vi "Bead threshold manual adjust.vi"(8 "error in (no error)":errorcluster, 9 "Range":cluster{"Lower value":sgl, "Upper value":sgl}={"Lower value"=40.0, "Upper value"=255.0}, 10 "Particle Filter Image":T1, 11 "Image Source":T1) -> (0 "error out":errorcluster, 3 "Refnum out":T1)   [LabVIEW 2020]
uses:
  <vilib>/vision/Image Controls.llb/IMAQ Image.ctl
  <vilib>/vision/NI_Vision_Development_Module.lvlib
panel:
  in  "stop":bool
  in  "Horizontal Pointer Slide":cluster{dbl, dbl}(slide)={0.0, 8.181818181818182} scale=0.0..255.0
  out "Source Imahe":T1(plugin-control) caption="Threshold Image"
  out "Threshold":T1(plugin-control) caption="Threshold Image"
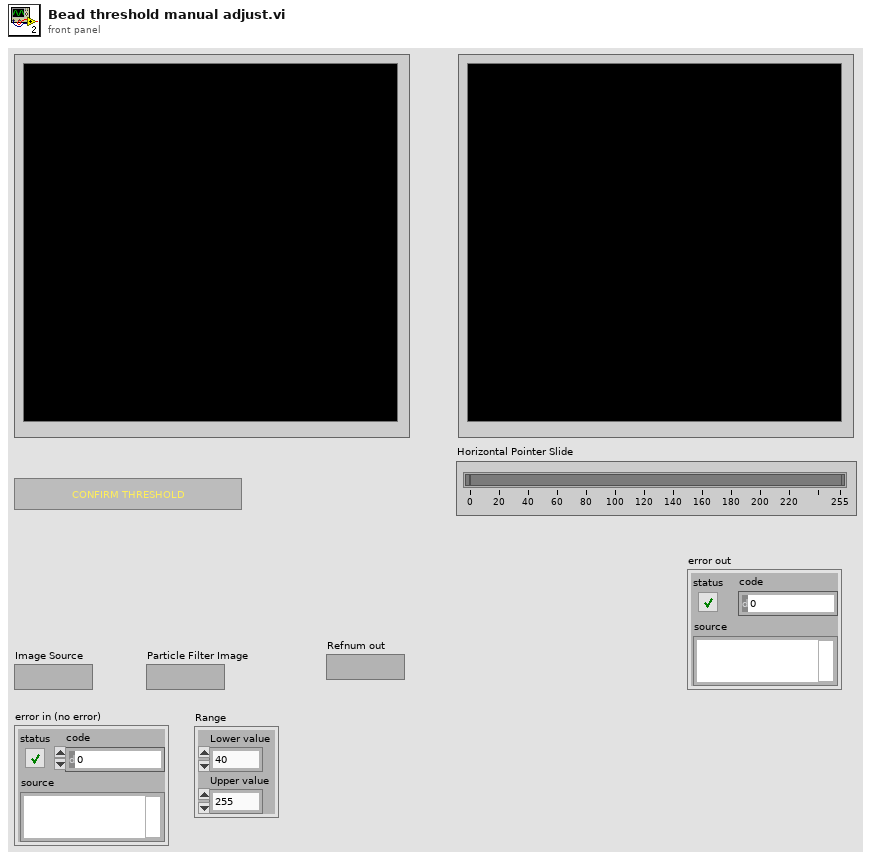
[diagram p1: front panel]
types:
  T1 = typedef "IMAQ Image.ctl" = refnum<image>
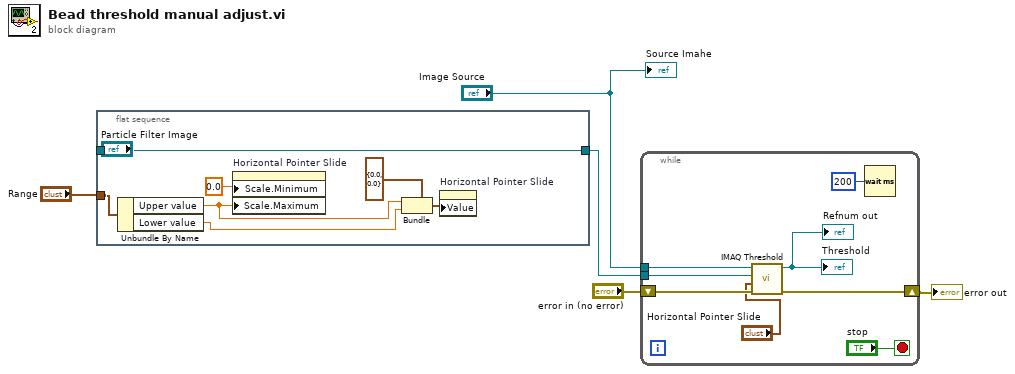
[diagram p0: block diagram]
diagram:
  n1 = flat-sequence {
    tunnel: "Particle Filter Image" -> [w12]
    tunnel: "Range" -> [w13]
    tunnel: [w12] -> w1
    frame #0 {
      n2 = Unbundle By Name(w13) -> ("Upper value"=w7:sgl, "Lower value"=w11:sgl)
      n3 = property on="Horizontal Pointer Slide" class="Slide (strict)"("Scale.Minimum"=0.0 ("Scale.Range:Maximum"), "Scale.Maximum"=w7) -> ()  [unwired: 2 in, 2 out]
      n4 = Bundle(cluster=cluster{dbl, dbl} {0.0, 0.0} ("Horizontal Pointer Slide"), w7, w11) -> (w9:cluster{dbl, dbl})
      n5 = property on="Horizontal Pointer Slide" class="Slide (strict)"("Value"=w9) -> ()  [unwired: 2 in, 2 out]
    }
  }
  n6 = while {
    tunnel: "Image Source" -> [w18]
    tunnel: w1 -> [w17]
    shift-right: [w20] -> w5
    shift-left: "error in (no error)" -> [w21]
    stop <- "stop" stop-if-true
    n7 = call "IMAQ Threshold"("error in (no error)"=w21, "Range"="Horizontal Pointer Slide", "Image Dst"=w17, "Image Src"=w18) -> ("error out"=w20:errorcluster, "Image Dst Out"=→"Refnum out" →"Threshold":T1)  [unwired: 6 in]
    n8 = Wait (ms)(milliseconds to wait=u32 200) -> ()  [unwired: 1 out]
  }
  "error out" <- w5
  "Source Imahe" <- "Image Source"
